vi "Initialize.vi"(7 "not in use":string="Setpoint.ch%d.SP", 8 "error in":errorcluster, 9 "Number of Channels":u32=1, 10 "Instance Name":string="PluginName", 11 "Voltage Setpoint in":refnum<class "Voltage Setpoint.lvclass">) -> (0 "error out":errorcluster, 3 "Voltage Setpoint out":refnum<class "Voltage Setpoint.lvclass">)   [LabVIEW 2023, in "Voltage Setpoint.lvclass"]
uses:
  Voltage Setpoint.lvclass
  Parents/Setpoint/Setpoint.lvclass
  Voltage Setpoint.lvclass/Voltage Setpoint.ctl
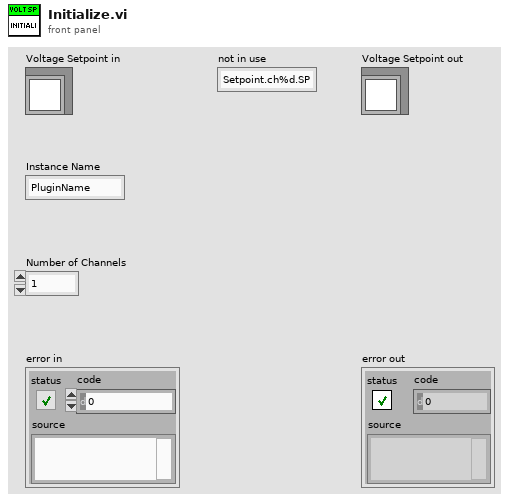
[diagram p1: front panel]
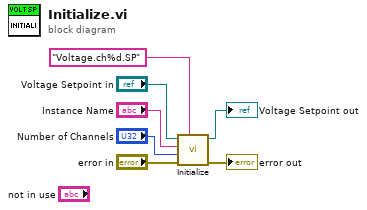
[diagram p0: block diagram]
diagram:
  n1 = call-parent "Initialize.vi"("ChannelName"="Voltage.ch%d.SP", "error in"="error in", "Number of Channels"="Number of Channels", "Instance Name"="Instance Name", "Setpoint in"="Voltage Setpoint in") -> ("error out"=→"error out":errorcluster, "Setpoint out"=→"Voltage Setpoint out":refnum<class "Voltage Setpoint.lvclass">)  [unwired: 5 in]
